vi "reprTextual.vi"(8 "error in (no error)":errorcluster, 11 "Idle in":refnum<class "Idle.lvclass">) -> (0 "error out":errorcluster, 2 "Description":string, 3 "Idle out":refnum<class "Idle.lvclass">)   [LabVIEW 2011, in "Idle.lvclass"]
doc: "Returns a string that represents what the mission does."
uses:
  Idle.lvclass
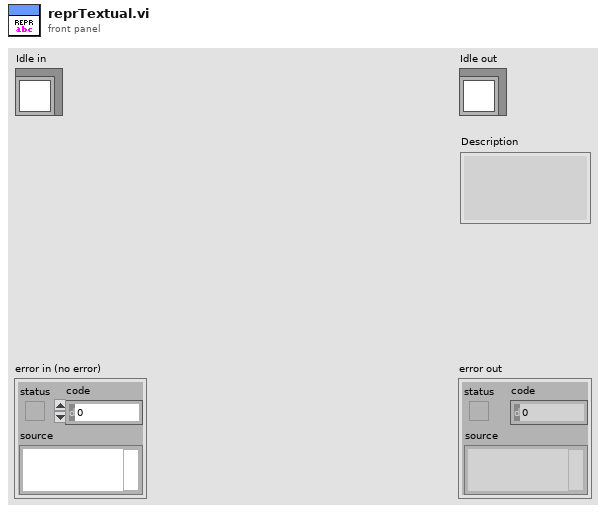
[diagram p1: front panel]
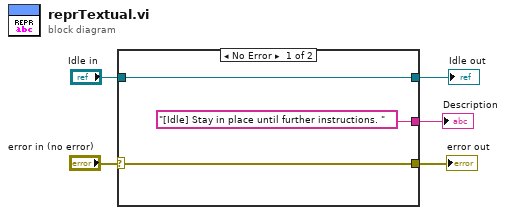
[diagram p0: block diagram]
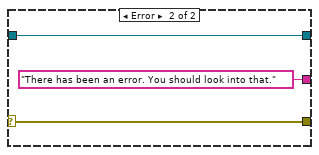
[diagram p2: hidden frame]
diagram:
  n1 = case shown="No Error" "error in (no error)" {
    selector: "error in (no error)" -> [w7 w10]
    tunnel: ["[Idle] Stay in place until further instructions. " "There has been an error. You should look into that."] -> w4
    tunnel: [w7 w10] -> w3
    tunnel: "Idle in" -> [w6 w9]
    tunnel: [w6 w9] -> w1
    frame No Error {
    }
    frame Error {
    }
  }
  "error out" <- w3
  "Idle out" <- w1
  "Description" <- w4
